vi "Periodic Tasks.vi"(8 "error in":errorcluster) -> ()   [LabVIEW 2025]
doc: "This VI runs in parallel to other robot code. It can contain as many user-defined periodic loops as you need. These can carry out PID or other sorts of timed response."
uses:
  <vilib>/Analysis/coordinate.llb/Angle Units.ctl
  <vilib>/Rock Robotics/WPI/DriverStation/WPI_DriverStationAllianceInfo.ctl
  <vilib>/Analysis/coordinate.llb/Wrap Angle (scalar).vi
  <vilib>/Rock Robotics/WPI/ThirdParty/Phoenix-LabVIEW/Pigeon IMU/CTRE_PigeonIMU_GetYPR.vi
  Robot Global Data.vi
  <vilib>/Rock Robotics/Network Tables/NT Write Number.vi
  <vilib>/Rock Robotics/Network Tables/NT Write Numeric Array.vi
  <vilib>/Rock Robotics/Network Tables/NT Write Boolean.vi
  <vilib>/Rock Robotics/Network Tables/NT Write String.vi
  <vilib>/Analysis/NI_AAL_Angle.lvlib
panel:
  out "s? t:f":T1
  in  "output cluster":T1
  out "error out":errorcluster
  out "error out 2":errorcluster
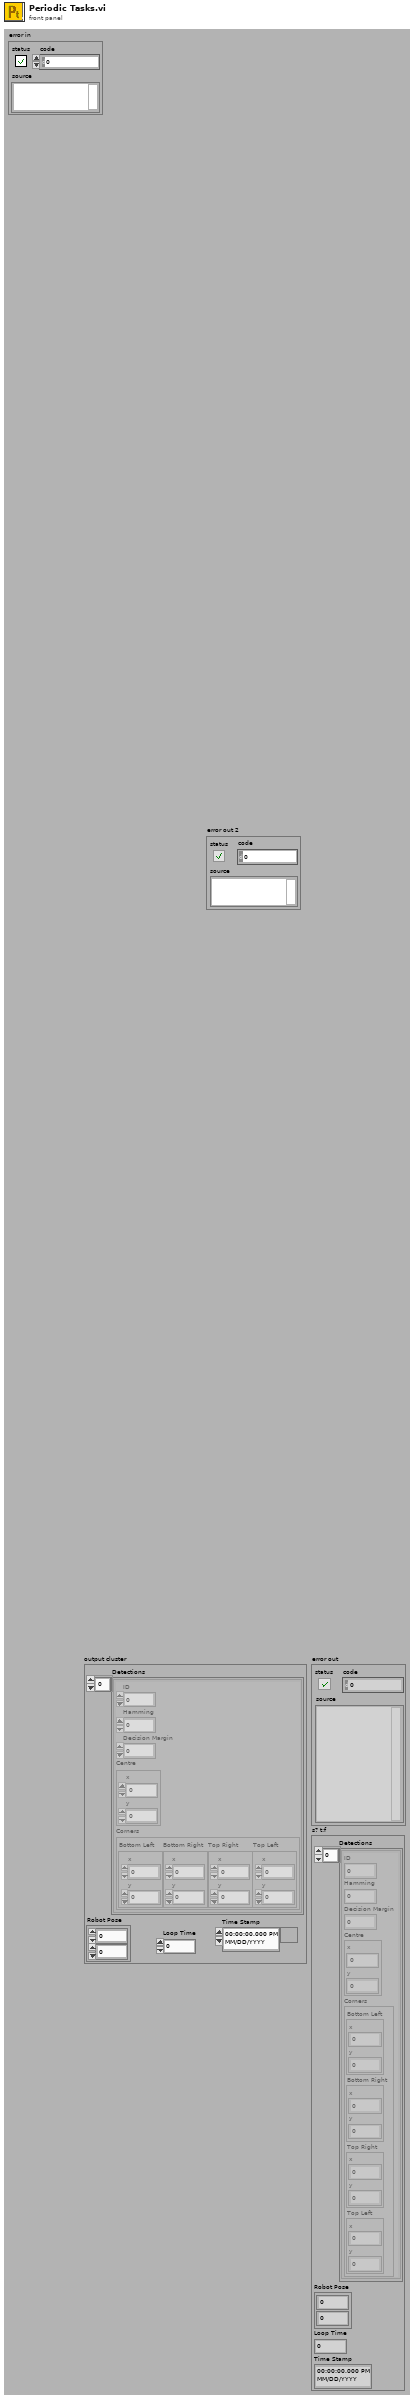
[diagram p1: front panel]
types:
  T1 = cluster{"Detections":cluster{"ID":i32, "Hamming":i32, "Decision Margin":sgl, "Centre":cluster{"x":dbl, "y":dbl}, "Corners":cluster{"Bottom Left":cluster{"x":dbl, "y":dbl}, "Bottom Right":cluster{"x":dbl, "y":dbl}, "Top Right":cluster{"x":dbl, "y":dbl}, "Top Left":cluster{"x":dbl, "y":dbl}}}[], "Robot Pose":cluster{dbl, dbl}, "Loop Time":dbl, "Time Stamp":timestamp}
  T2 = typedef "WPI_DriverStationAllianceInfo.ctl" = enum16{"Red", "Blue", "Invalid"}
  T3 = typedef "NI_AAL_Angle.lvlib/Angle Units.ctl" = i32
  T4 = typedef "WPI_DriverStationRobotMode2.ctl" = enum16{"Autonomous Disabled", "Autonomous Enabled", "Teleop Disabled", "Teleop Enabled", "Disconnected", "Finish", "Test Disabled", "Test Enabled", "Emergency Stopped"}
  T5 = typedef "CTRE_PigeonIMU_DeviceRef.ctl" = cluster{"DeviceStatus":errorcluster, "Device Number":u8, "Type":T6, "Device ID":u32, "Handle":u64, "UsageFrame":u32, "Library Path":path}
  T6 = typedef "CTRE_PigeonIMU_ConnectionType.ctl" = u32
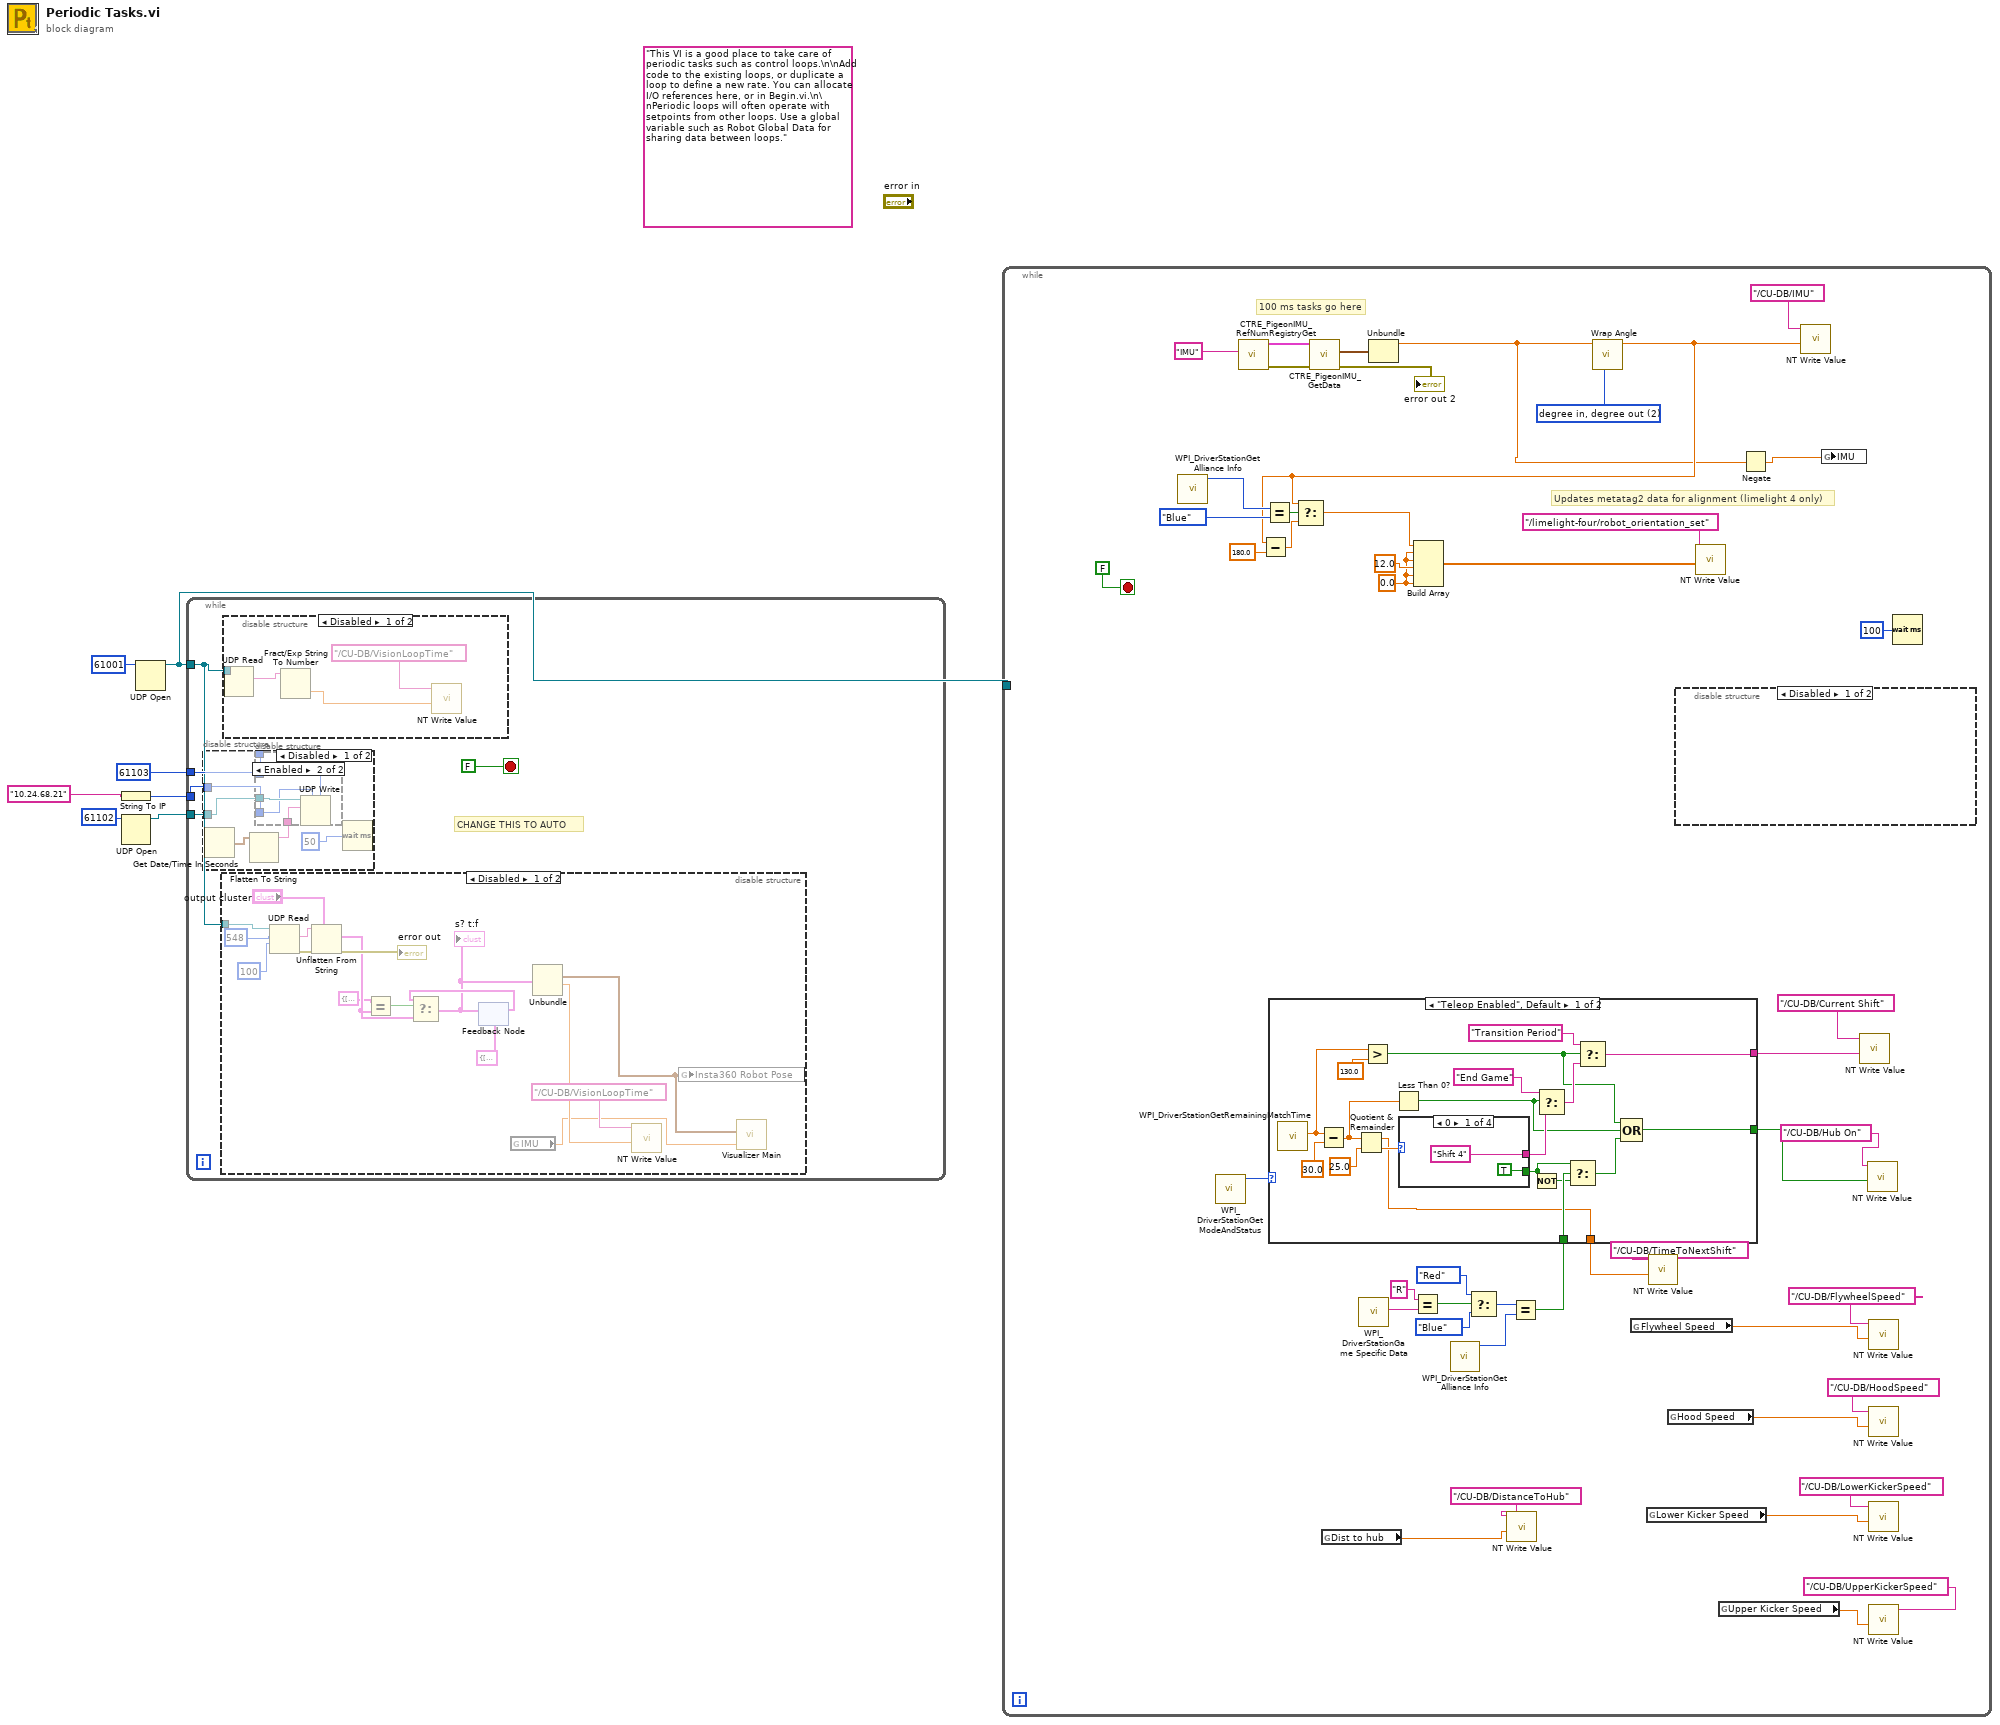
[diagram p0: block diagram]
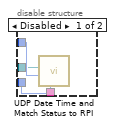
[diagram p2: hidden frame]
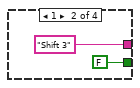
[diagram p7: hidden frame]
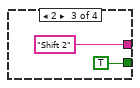
[diagram p8: hidden frame]
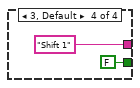
[diagram p9: hidden frame]
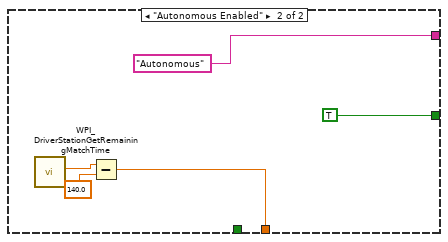
[diagram p10: hidden frame]
diagram:
  (unwired) "This VI is a good place to take care of periodic tasks such as control loops.\n\nAdd code to the existing loops, or duplicate a loop to define a new rate. You can allocate I/O references here, or in Begin.vi.\n\nPeriodic loops will often operate with setpoints from other loops. Use a global variable such as Robot Global Data for sharing data between loops."
  n1 = String To IP(1:"10.24.68.21" ("name")) -> (0:w4:u32)
  n2 = UDP Open(11:u16 61102 ("port")) -> (port=w2:refnum<k16>)  [unwired: 4 in, 2 out]
  n3 = UDP Open(11:u16 61001 ("port")) -> (port=w1:refnum<k16>)  [unwired: 4 in, 2 out]
  n4 = while {
    tunnel: w1 -> [w8]
    tunnel: w4 -> [w11]
    tunnel: u16 61103 -> [w10]
    tunnel: w2 -> [w9]
    stop <- FALSE stop-if-true
    # "CHANGE THIS TO AUTO"
    n5 = disable-structure shown="Disabled" {
      disable-tunnel: w11 -> [w18 _]
      disable-tunnel: w10 -> [w17 _]
      disable-tunnel: w9 -> [w16 _]
      frame Disabled {
        n6 = Get Date/Time In Seconds() -> (seconds since 1Jan1904=w14:timestamp)
        n7 = Flatten To String(anything=w14) -> (data string=w13:string)  [unwired: 3 in, 2 out]
        n8 = disable-structure shown="Enabled" {
          disable-tunnel: w18 -> [w21 w23]
          disable-tunnel: w17 -> [w20 w24]
          disable-tunnel: w16 -> [w19 w25]
          disable-tunnel: w13 -> [_ w22]
          frame Disabled {
            n9 = call "UDP Date Time and Match Status to RPI.vi"("Address"=w21, "Port"=w20, "port"=w19) -> ()  [unwired: 9 in]
          }
          frame Enabled {
            n10 = UDP Write(address=w23, port or service name=w24, connection ID=w25, data in=w22) -> ()  [unwired: 2 in, 2 out]
          }
        }
        n11 = Wait (ms)(milliseconds to wait=u32 50) -> ()  [unwired: 1 out]
      }
      frame Enabled {
      }
    }
    n12 = disable-structure shown="Disabled" {
      disable-tunnel: w8 -> [w27 _]
      frame Disabled {
        n13 = UDP Read(connection ID=w27, max size (548)=548, timeout ms (25000)=100) -> (data out=w41:string, error out=w40:errorcluster)  [unwired: 1 in, 3 out]
        n14 = Unflatten From String(type="output cluster", binary string=w41, error in (no error)=w40) -> (value=w34:T1, error out=→"error out":errorcluster)  [unwired: 2 in, 1 out]
        n15 = Equal?(x=T1 {"Detections"=[], "Robot Pose"={0.0, 0.0}, "Loop Time"=0.0, "Time Stamp"=timestamp(0 s since 1904-01-01)}, y=w34) -> (x = y?=w37:bool)
        n16 = feedback #1(T1 {"Detections"=[], "Robot Pose"={0.0, 0.0}, "Loop Time"=0.0, "Time Stamp"=timestamp(0 s since 1904-01-01)} ("output cluster")) -> (w36:T1)
        n17 = Select(t=w36, s=w37, f=w34) -> (s? t:f=w28:T1)
        "s? t:f" <- w28
        n18 = feedback-in #1(w28) -> ()
        n19 = global read "Robot Global Data.vi" "IMU"() -> (w26:dbl)
        n20 = Unbundle(w28) -> ("Robot Pose"=w31:cluster{dbl, dbl}, "Loop Time"=w32:dbl)  [unwired: 2 out]
        n21 = call-poly <vilib>:"NT Write Value.vi"("value"=w32, "name"="/CU-DB/VisionLoopTime") -> ()  [unwired: 9 in, 1 out]
        n22 = global write "Robot Global Data.vi" "Insta360 Robot Pose"(w31) -> ()
        n23 = call "Visualizer Main.vi"("Theta"=w26, "Insta360 Pose"=w31) -> ()  [unwired: 10 in]
      }
      frame Enabled {
      }
    }
    n24 = disable-structure shown="Disabled" {
      disable-tunnel: w8 -> [w46 _]
      frame Disabled {
        n25 = UDP Read(connection ID=w46) -> (data out=w45:string)  [unwired: 3 in, 4 out]
        n26 = Fract/Exp String To Number(string=w45) -> (number=w44:dbl)  [unwired: 3 in, 1 out]
        n27 = call-poly <vilib>:"NT Write Value.vi"("value"=w44, "name"="/CU-DB/VisionLoopTime") -> ()  [unwired: 9 in, 1 out]
      }
      frame Enabled {
      }
    }
  }
  n28 = while {
    tunnel: w1 -> [_]
    stop <- FALSE stop-if-true
    w84 = 0.0 ("element")
    w88 = T3 2 items=["radian in, radian out", "radian in, degree out", "degree in, degree out", "degree in, radian out"] ("angle units")
    # "Updates metatag2 data for alignment (limelight 4 only)"
    # "100 ms tasks go here"
    n29 = call <vilib>:"WPI_DriverStationGet Alliance Info.vi"() -> ("Alliance"=w81:T2)  [unwired: 6 in, 5 out]
    n30 = call <vilib>:"WPI_DriverStationGetModeAndStatus.vi"() -> ("Robot Mode"=w64:T4)  [unwired: 10 in, 1 out]
    n31 = call <vilib>:"CTRE_PigeonIMU_RefNumRegistryGet.vi"("refnum name"="IMU") -> ("error out"=w92:errorcluster, "PigeonIMUDevRef"=w91:T5)  [unwired: 9 in]
    n32 = Equal?(x=w81, y=WPI_DriverStationAllianceInfo."Blue") -> (x = y?=w79:bool)
    n33 = call-poly <vilib>:"CTRE_PigeonIMU_GetData.vi"("error in (no error)"=w92, "PigeonIMUDevRef"=w91) -> ("error out"=→"error out 2":errorcluster, "Yaw Pitch Roll"=w87:cluster{"Yaw":dbl, "Pitch":dbl, "Roll":dbl})  [unwired: 7 in, 1 out]
    n34 = global read "Robot Global Data.vi" "Dist to hub"() -> (w50:dbl)
    n35 = call <vilib>:"WPI_DriverStationGame Specific Data.vi"() -> ("Game Specific Data"=w62:string)  [unwired: 11 in]
    n36 = Unbundle(w87) -> ("Yaw"=w47:dbl)  [unwired: 2 out]
    n37 = Equal?(x="R", y=w62) -> (x = y?=w63:bool)
    n38 = call <vilib>:"WPI_DriverStationGet Alliance Info.vi"() -> ("Alliance"=w60:T2)  [unwired: 6 in, 5 out]
    n39 = Select(t=WPI_DriverStationAllianceInfo."Red" ("Alliance"), s=w63, f=WPI_DriverStationAllianceInfo."Blue") -> (s? t:f=w59:T2)
    n40 = call-poly <vilib>:"NT Write Value.vi"("value"=w50, "name"="/CU-DB/DistanceToHub") -> ()  [unwired: 9 in, 1 out]
    n41 = Equal?(x=w59, y=w60) -> (x = y?=w58:bool)
    n42 = case shown="\"Teleop Enabled\", Default" w64 {
      tunnel: [w111 "Autonomous"] -> w61
      tunnel: w58 -> [w101 _]
      tunnel: [w95 TRUE] -> w57
      tunnel: [w94 w121] -> w52
      frame "Teleop Enabled", Default {
        n43 = call <vilib>:"WPI_DriverStationGetRemainingMatchTime.vi"() -> ("Match Time(s)"=w102:sgl)  [unwired: 10 in, 1 out]
        n44 = Subtract(x=w102, y=sgl 30.0) -> (x-y=w105:sgl)
        n45 = Quotient & Remainder(x=w105, y=sgl 25.0) -> (x-y*floor(x/y)=w94:sgl, floor(x/y)=w104:sgl)
        n46 = Greater?(x=w102, y=130.0) -> (0:w96:bool)
        n47 = Less Than 0?(x=w105) -> (x < 0?=w97:bool)
        n48 = case shown="0" w104 {
          tunnel: ["Shift 4" "Shift 3" "Shift 2" "Shift 1"] -> w103
          tunnel: [TRUE FALSE TRUE FALSE] -> w99
          frame 0 {
          }
          frame 1 {
          }
          frame 2 {
          }
          frame 3, Default {
          }
        }
        n49 = Not(x=w99) -> (.not. x?=w100:bool)
        n50 = Select(t="End Game", s=w97, f=w103) -> (s? t:f=w109:string)
        n51 = Select(t=w99, s=w101, f=w100) -> (s? t:f=w98:bool)
        n52 = Select(t="Transition Period", s=w96, f=w109) -> (s? t:f=w111:string)
        n53 = Compound Arithmetic op=OR(w96, w97, w98) -> (w95:bool)
      }
      frame "Autonomous Enabled" {
        n54 = call <vilib>:"WPI_DriverStationGetRemainingMatchTime.vi"() -> ("Match Time(s)"=w123:sgl)  [unwired: 10 in, 1 out]
        n55 = Subtract(x=w123, y=sgl 140.0) -> (x-y=w121:sgl)
      }
    }
    n56 = call-poly <vilib>:"Wrap Angle.vi"("angle units"=w88, "angle in"=w47) -> ("angle out"=w78:dbl)  [unwired: 8 in, 1 out]
    n57 = Subtract(x=w78, y=180.0) -> (x-y=w77:dbl)
    n58 = Select(t=w78, s=w79, f=w77) -> (s? t:f=w76:dbl)
    n59 = Build Array(w76, w84, w84, 12.0 ("element"), w84, w84) -> (w86:dbl[])
    n60 = global read "Robot Global Data.vi" "Flywheel Speed"() -> (w56:dbl)
    n61 = global read "Robot Global Data.vi" "Lower Kicker Speed"() -> (w54:dbl)
    n62 = call-poly <vilib>:"NT Write Value.vi"("value"=w52, "name"="/CU-DB/TimeToNextShift") -> ()  [unwired: 9 in, 1 out]
    n63 = global read "Robot Global Data.vi" "Hood Speed"() -> (w53:dbl)
    n64 = disable-structure shown="Disabled" {
      frame Disabled {
      }
      frame Enabled {
      }
    }
    n65 = call-poly <vilib>:"NT Write Value.vi"("value"=w86, "name"="/limelight-four/robot_orientation_set") -> ()  [unwired: 9 in, 1 out]
    n66 = global read "Robot Global Data.vi" "Upper Kicker Speed"() -> (w55:dbl)
    n67 = Negate(x=w47) -> (-x=w48:dbl)
    n68 = call-poly <vilib>:"NT Write Value.vi"("value"=w78, "name"="/CU-DB/IMU") -> ()  [unwired: 9 in, 1 out]
    n69 = global write "Robot Global Data.vi" "IMU"(w48) -> ()
    n70 = call-poly <vilib>:"NT Write Value.vi"("value"=w61, "name"="/CU-DB/Current Shift") -> ()  [unwired: 9 in, 1 out]
    n71 = call-poly <vilib>:"NT Write Value.vi"("value"=w57, "name"="/CU-DB/Hub On") -> ()  [unwired: 9 in, 1 out]
    n72 = call-poly <vilib>:"NT Write Value.vi"("value"=w56, "name"="/CU-DB/FlywheelSpeed") -> ()  [unwired: 9 in, 1 out]
    n73 = call-poly <vilib>:"NT Write Value.vi"("value"=w53, "name"="/CU-DB/HoodSpeed") -> ()  [unwired: 9 in, 1 out]
    n74 = call-poly <vilib>:"NT Write Value.vi"("value"=w54, "name"="/CU-DB/LowerKickerSpeed") -> ()  [unwired: 9 in, 1 out]
    n75 = call-poly <vilib>:"NT Write Value.vi"("value"=w55, "name"="/CU-DB/UpperKickerSpeed") -> ()  [unwired: 9 in, 1 out]
    n76 = Wait (ms)(milliseconds to wait=u32 100) -> ()  [unwired: 1 out]
  }
